vi "libdaq_device_setUID_byindex.vi"(0 "error in (no error)":errorcluster, 3 "device_index":u32, 5 "UID state":bool=TRUE) -> (14 "error out":errorcluster)   [LabVIEW 2010, in "libdaqVI.lvlib"]
doc: "设置设备的UID指示灯状态，当控制系统连接多个DAQ设备时，找到特定的某个DAQ设备有时会比较困难，因此通过点亮特定设备的UID指示灯可以快速的定位到该设备"
uses:
  libdaqVI.lvlib
  dll/daqlib.dll
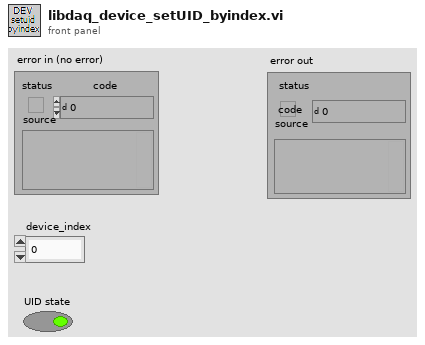
[diagram p1: front panel]
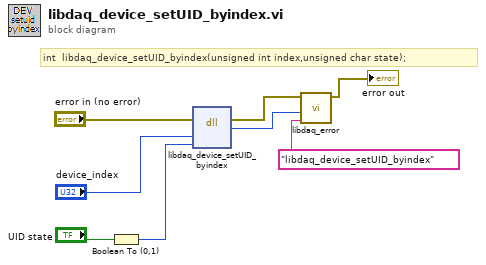
[diagram p0: block diagram]
diagram:
  # "int  libdaq_device_setUID_byindex(unsigned int index,unsigned char state);"
  n1 = Boolean To (0,1)(Boolean="UID state") -> (0, 1=w5:i16)
  n2 = dll-call lib="E:/Product/Example/DAQ-USB3212/Labview/labview_2010/libdaqVI/dll/daqlib.dll" fn="libdaq_device_setUID_byindex"(error in="error in (no error)", "device_index"="device_index", "state"=w5) -> (error out=w4:errorcluster, "return type"=w2:i32)  [unwired: 4 in, 1 out]
  n3 = call "libdaq_error.vi"("error source"="libdaq_device_setUID_byindex", "error code"=w2, "错误输入（无错误）"=w4) -> ("错误输出"=→"error out":errorcluster)  [unwired: 8 in]
